vi "svl_Waterfall Display.vi"() -> ()   [LabVIEW 2017]
uses:
  <vilib>/addons/Sound and Vibration/compatibility/Waterfall/subVIs/svl_Waterfall Global.vi
panel:
  in  "palette":T1={"x axis width [%]"=80.0, "z axis height [%]"=40.0, "autoscale x"=FALSE, "autoscale y"=FALSE, "autoscale z max"=FALSE, "autoscale all"=FALSE, "transparency"=FALSE, "store view"=FALSE, "restore view"=FALSE} {"x axis width [%]" min=10.0 max=100.0 step=1.0 scale=10.0..100.0 scale format="%.1f"; "z axis height [%]" min=10.0 max=99.99 step=1.0 scale=10.0..100.0 scale format="%.1f"}
  in  "stop":bool
  in  "y axis":dbl(slide)=1234.0 scale=0.0..50.0 scale format="%.1f"
  in  "z axis":dbl(slide) scale format="%.1f"
  in  "x axis":dbl(slide) scale=0.0..30000.0 scale format="%.1f"
  out "Graph":cluster{dbl[], dbl[]}[](graph)
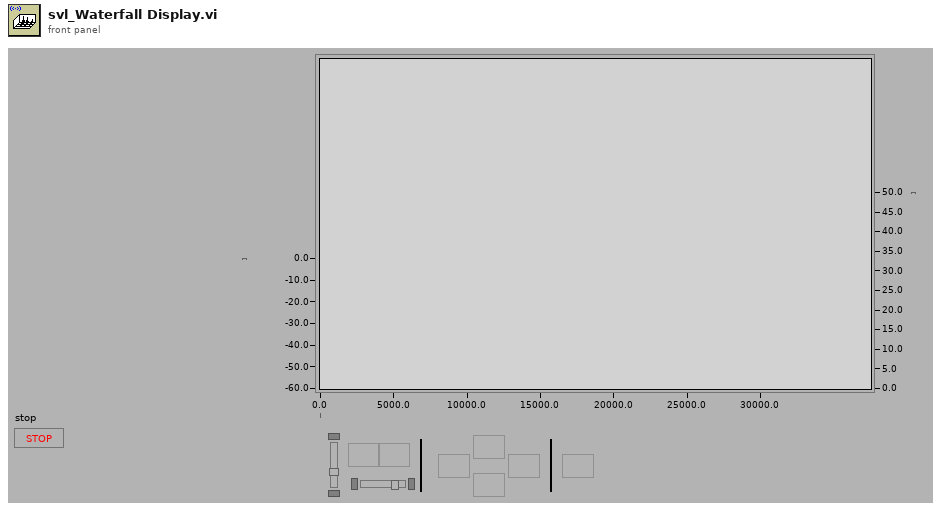
[diagram p1: front panel]
types:
  T1 = cluster{"x axis width [%]":dbl, "z axis height [%]":dbl, "autoscale x":bool, "autoscale y":bool, "autoscale z max":bool, "autoscale all":bool, "transparency":bool, "store view":bool, "restore view":bool}
  T2 = cluster{"autoscale x":bool, "autoscale y":bool, "autoscale z":bool, "autoscale all":bool, "transparency":bool, "store view":bool, "restore view":bool}
  T3 = cluster{"x axis width [%]":dbl, "z axis height [%]":dbl, "x axis minimum":dbl, "x axis maximum":dbl, "z axis minimum":dbl, "z axis maximum":dbl, "y axis minimum":dbl, "y axis maximum":dbl}
  T4 = typedef "LVPositionTypeDef.ctl" = cluster{"Left":i32, "Top":i32}
  T5 = cluster{"x axis width [%]":dbl, "z axis height [%]":dbl, "Scale.Minimum":dbl, "Scale.Maximum":dbl, "Scale.Minimum":dbl, "Scale.Maximum":dbl, "Scale.Minimum":dbl, "Scale.Maximum":dbl}
  T6 = cluster{"autoscale x":bool, "autoscale y":bool, "autoscale z max":bool, "autoscale all":bool, "transparency":bool, "store view":bool, "restore view":bool}
  T7 = cluster{"x axis width [%]":bool, "z axis height [%]":bool, bool, bool, bool, bool, bool, bool}
  T8 = cluster{"autoscale x":bool, "autoscale y":bool, bool, "autoscale all":bool, "transparency":bool, "store view":bool, "restore view":bool}
  T9 = cluster{"x axis width [%]":dbl, "z axis height [%]":dbl, "Scale.Minimum":dbl, "Scale.Maximum":dbl, "Scale.Minimum":dbl, "Scale.Maximum":dbl, "Scale.Minimum":dbl, "Scale.Maximum":dbl, "transparency":bool}
  T10 = cluster{"x axis":string, "y axis":string, "z axis":string}
  T11 = cluster{"Scale.Minimum":dbl, "Scale.Maximum":dbl}
  T12 = cluster{"y index":i32, "y length":i32, "x index":i32, "x length":i32}
  T13 = cluster{"frame":u32, "plot":u32, "background":u32}
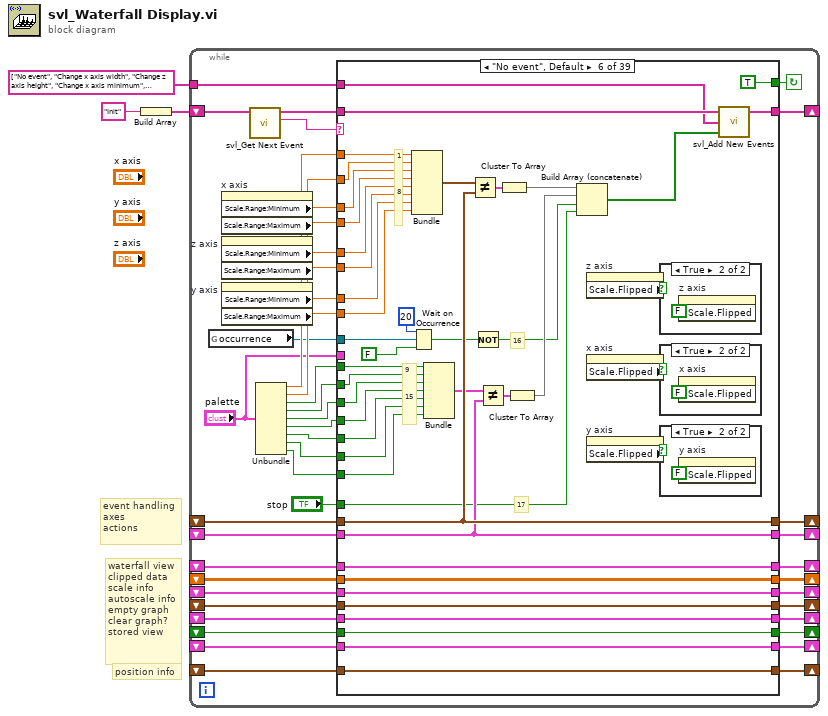
[diagram p0: block diagram]
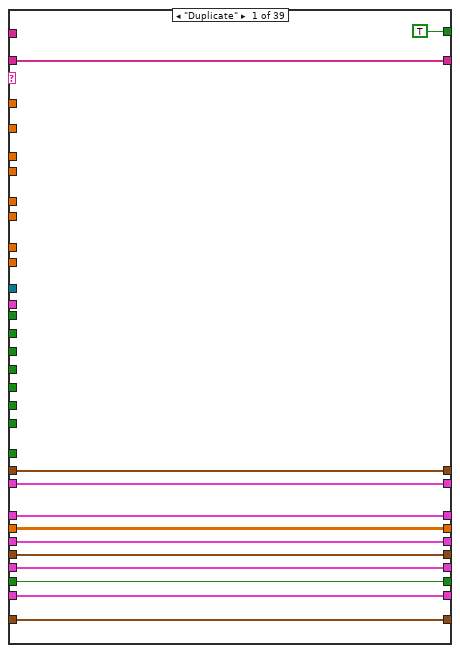
[diagram p2: hidden frame]
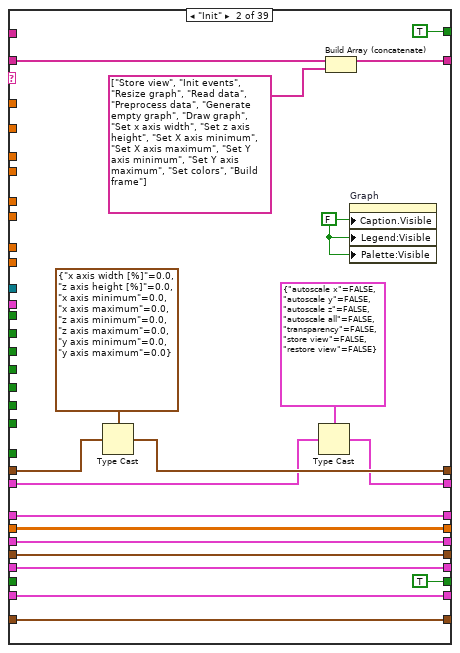
[diagram p3: hidden frame]
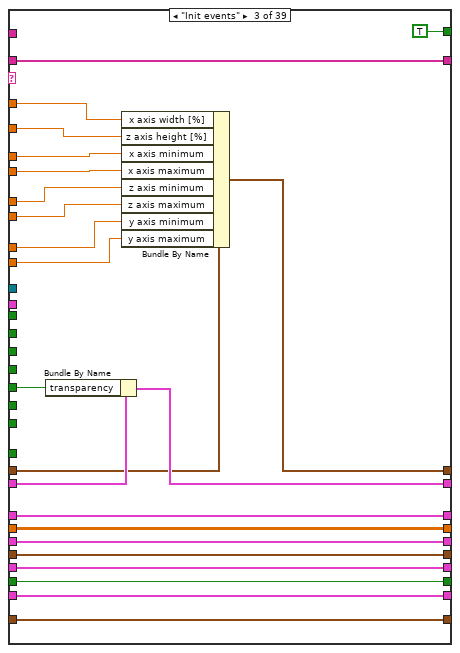
[diagram p4: hidden frame]
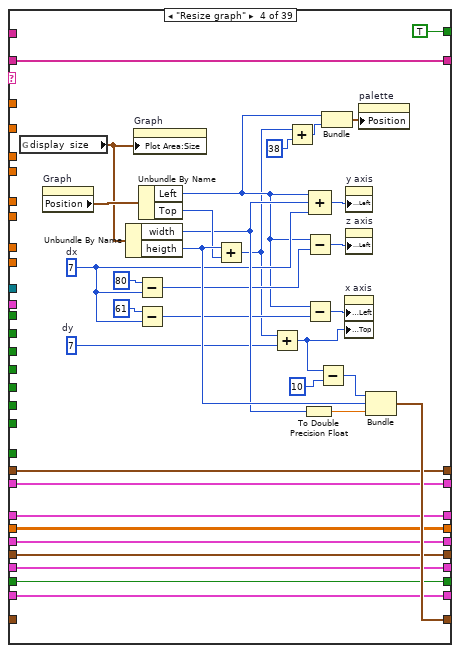
[diagram p5: hidden frame]
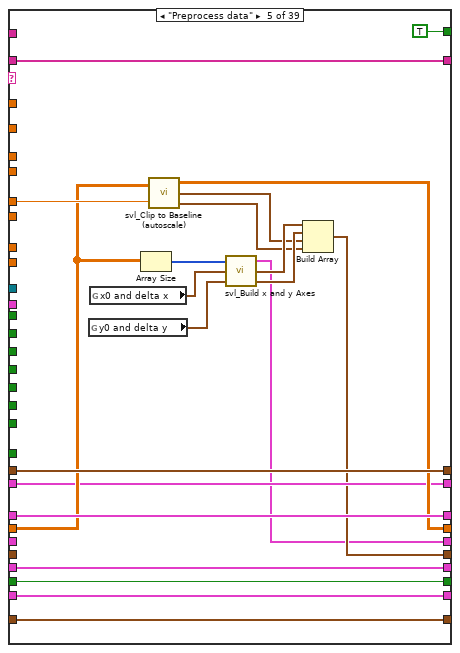
[diagram p6: hidden frame]
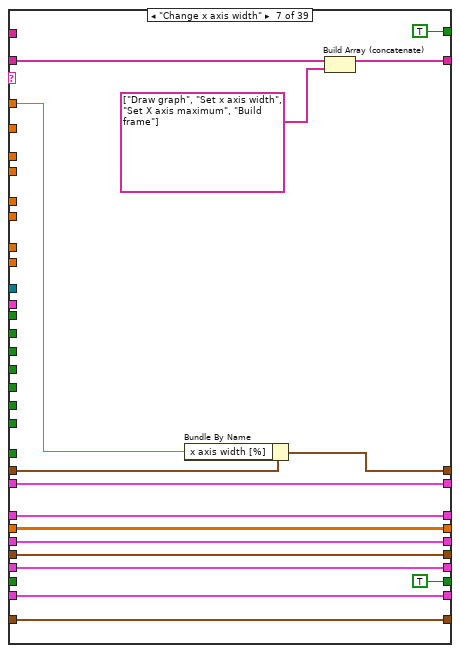
[diagram p10: hidden frame]
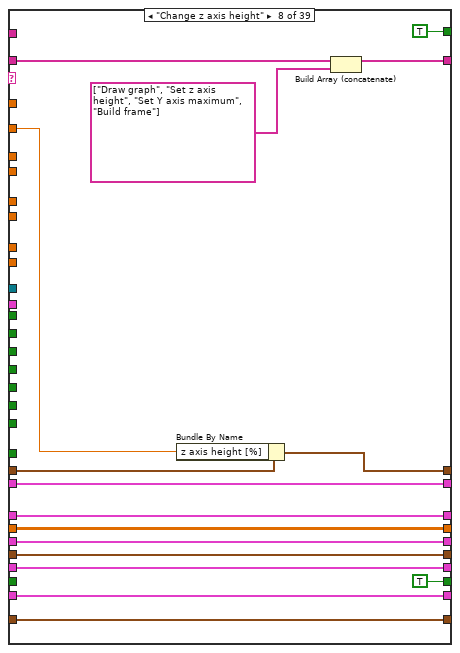
[diagram p11: hidden frame]
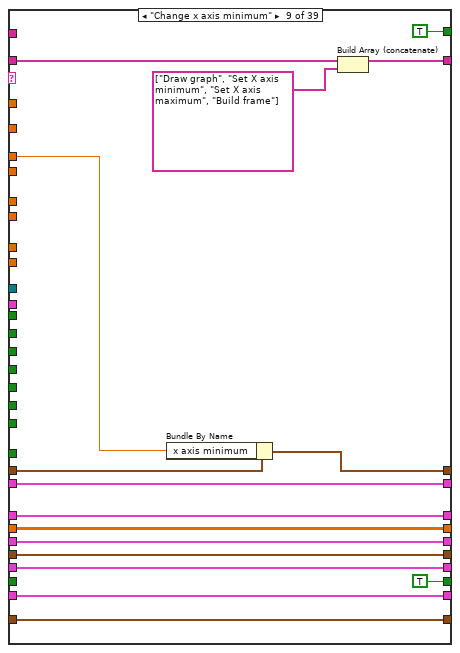
[diagram p12: hidden frame]
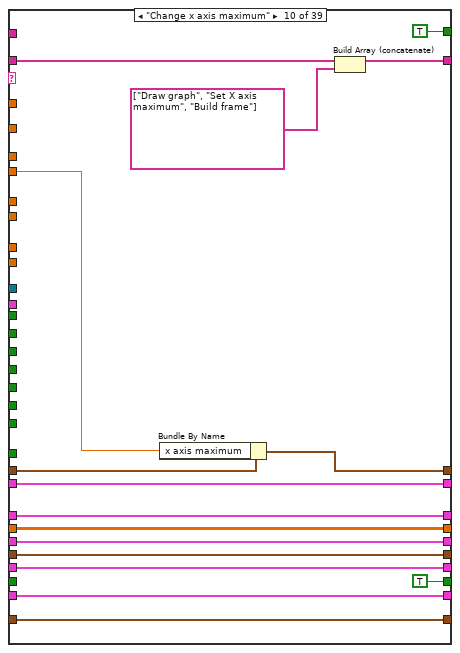
[diagram p13: hidden frame]
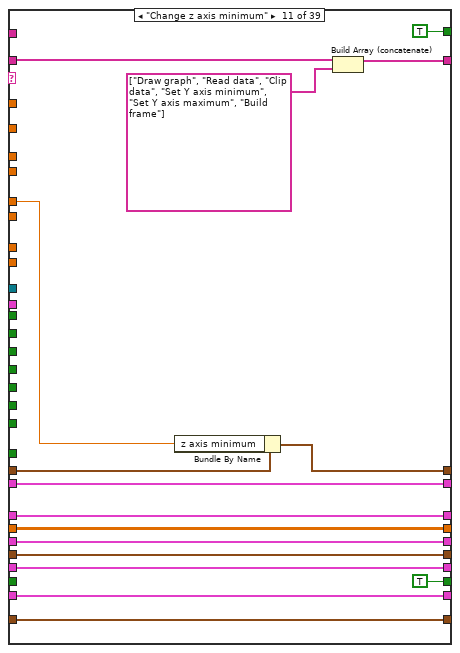
[diagram p14: hidden frame]
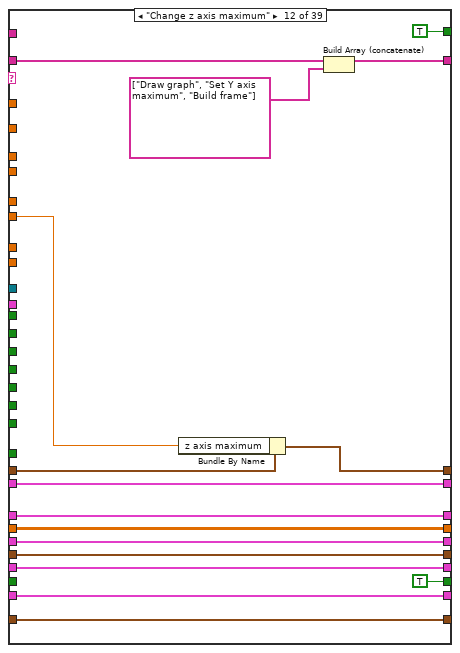
[diagram p15: hidden frame]
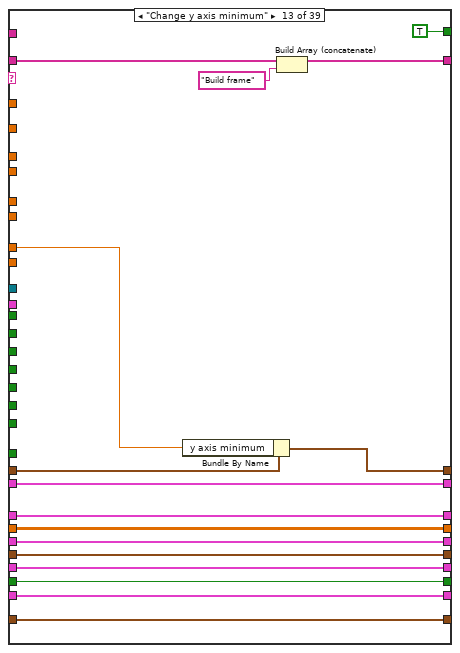
[diagram p16: hidden frame]
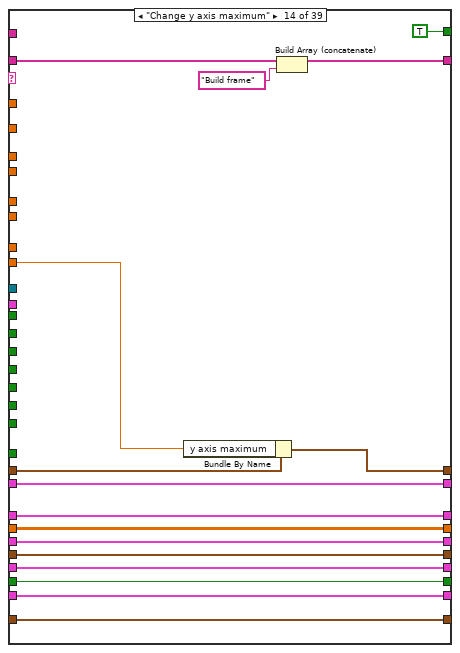
[diagram p17: hidden frame]
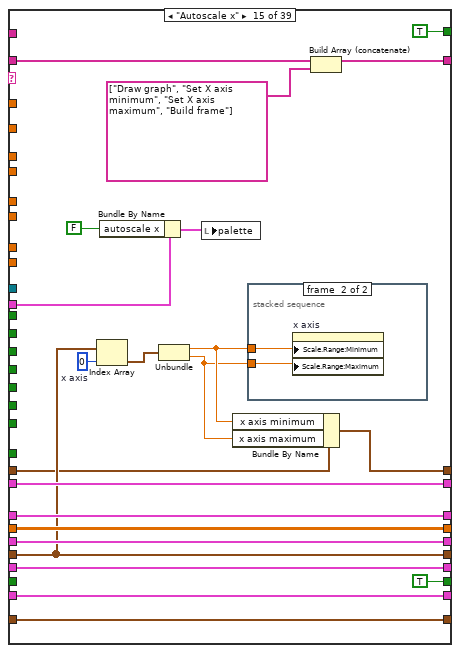
[diagram p18: hidden frame]
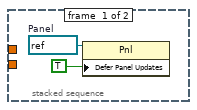
[diagram p19: hidden frame]
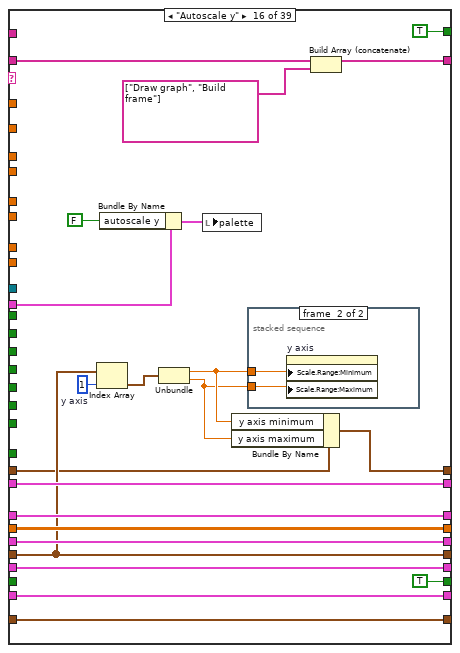
[diagram p20: hidden frame]
diagram:
  # "waterfall view\nclipped data\nscale info\nautoscale info\nempty graph\nclear graph?\nstored view"
  # "position info"
  # "event handling\naxes\nactions"
  n1 = Build Array("Init") -> (w2:string[])
  n2 = while {
    shift-left: _ -> [w16]
    shift-right: [w17] -> _
    shift-left: _ -> [w23]
    shift-right: [w22] -> _
    shift-left: _ -> [w25]
    shift-right: [w24] -> _
    shift-left: _ -> [w26]
    shift-right: [w27] -> _
    shift-left: _ -> [w29]
    shift-right: [w30] -> _
    shift-left: _ -> [w19]
    shift-right: [w32] -> _
    shift-left: _ -> [w31]
    shift-right: [w33] -> _
    shift-left: _ -> [w34]
    shift-right: [w35] -> _
    shift-left: _ -> [w38]
    shift-right: [w37] -> _
    shift-left: _ -> [w43]
    shift-right: [w44] -> _
    tunnel: string[] ["No event", "Change x axis width", "Change z axis height", "Change x axis minimum", "Change x axis maximum", "Change z axis minimum", "Change z axis maximum", "Change y axis minimum", "Change y axis maximum", "Autoscale x", "Autoscale y", "Autoscale z max", "Autoscale all", "Change transparency", "Store view", "Restore view", "Refresh", "Stop"] ("Event Names") -> [w46]
    shift-left: w2 -> [w21]
    shift-right: [w47] -> _
    stop <- w45 continue-if-true
    n3 = global read "svl_Waterfall Global.vi" "occurrence"() -> (w5:refnum<k4>)
    n4 = property on="x axis" class="Slide (strict)"() -> ("Scale.Range:Minimum"=w42:dbl, "Scale.Range:Maximum"=w41:dbl)  [unwired: 2 in, 2 out]
    n5 = property on="z axis" class="Slide (strict)"() -> ("Scale.Range:Minimum"=w40:dbl, "Scale.Range:Maximum"=w39:dbl)  [unwired: 2 in, 2 out]
    n6 = property on="y axis" class="Slide (strict)"() -> ("Scale.Range:Minimum"=w36:dbl, "Scale.Range:Maximum"=w28:dbl)  [unwired: 2 in, 2 out]
    n7 = call <vilib>:"svl_Get Next Event.vi"("Event Queue In"=w21) -> ("Next Event"=w4:string, "Event Queue Out"=w20:string[])  [unwired: 5 in]
    n8 = Unbundle("palette") -> ("x axis width [%]"=w15:dbl, "z axis height [%]"=w14:dbl, "autoscale x"=w7:bool, "autoscale y"=w8:bool, "autoscale z max"=w9:bool, "autoscale all"=w10:bool, "transparency"=w11:bool, "store view"=w12:bool, "restore view"=w13:bool)
    n9 = case shown="\"No event\", Default" w4 {
      tunnel: w20 -> [w58 w77 w93 w115 w156 w202 w220 w236 w251 w267 w283 w299 w306 w321 w343 w369 w393 w417 w433 w465 w474 w505 w526 w534 w570 w591 w631 w637 w654 w679 w696 w729 w751 w769 w800 w818 w823 w860 w887]
      tunnel: [w58 w76 w93 w115 w156 w201 w219 w222 w250 w254 w282 w298 w307 w322 w344 w360 w394 w418 w432 w465 w475 w504 w526 w534 w570 w591 w631 w637 w654 w679 w696 w729 w751 w769 w801 w818 w823 w860 w887] -> w47
      tunnel: w46 -> [_ _ _ _ _ w199 _ _ _ _ _ _ _ _ _ _ _ _ _ _ _ _ _ _ _ _ _ _ _ _ _ _ _ _ _ _ _ _ _]
      tunnel: [TRUE TRUE TRUE TRUE TRUE TRUE TRUE TRUE TRUE TRUE TRUE TRUE TRUE TRUE TRUE TRUE TRUE TRUE TRUE TRUE TRUE TRUE FALSE TRUE TRUE TRUE TRUE TRUE TRUE TRUE TRUE TRUE TRUE TRUE TRUE TRUE TRUE TRUE TRUE] -> w45
      tunnel: [w57 w72 w100 w125 w155 w197 w209 w225 w252 w268 w284 w300 w316 w332 w354 w380 w405 w425 w441 w464 w491 w513 w524 w556 w583 w602 w630 w648 w673 w690 w714 w728 w750 w768 w804 w817 w831 w871 w893] -> w44
      tunnel: w43 -> [w57 w72 w100 _ w155 w197 w209 w225 w252 w268 w284 w300 w316 w332 w354 w380 w405 w425 w441 w464 w491 w513 w524 w556 w583 w602 w630 w648 w673 w690 w714 w728 w750 w768 w804 w817 w831 w871 w893]
      tunnel: w15 -> [_ _ w84 _ _ w189 w210 _ _ _ _ _ _ _ _ _ _ _ _ w455 _ _ _ _ w578 _ _ _ w670 _ _ _ _ _ _ _ _ _ _]
      tunnel: w14 -> [_ _ w85 _ _ w196 _ w226 _ _ _ _ _ _ _ _ _ _ _ w454 _ _ _ _ _ w601 _ _ _ _ w707 _ _ _ w776 _ _ _ _]
      tunnel: w42 -> [_ _ w90 _ _ w195 _ _ w241 _ _ _ _ _ _ _ _ _ _ w453 _ _ _ _ _ _ _ w639 w672 _ _ _ _ _ w780 _ _ _ _]
      tunnel: w41 -> [_ _ w91 _ _ w190 _ _ _ w258 _ _ _ _ _ _ _ _ _ w452 _ _ _ _ _ _ _ _ w662 _ _ _ _ _ w774 _ _ _ _]
      tunnel: w40 -> [_ _ w89 _ w152 w194 _ _ _ _ w273 _ _ _ _ _ _ _ _ w451 _ _ _ _ _ _ _ _ _ w687 w706 _ w734 _ w778 _ _ _ _]
      tunnel: w39 -> [_ _ w88 _ _ w193 _ _ _ _ _ w291 _ _ _ _ _ _ _ w450 _ _ _ _ _ _ _ _ _ _ w705 _ _ _ w779 _ _ _ _]
      tunnel: [w56 w74 w80 w117 w154 w187 w218 w234 w242 w259 w276 w288 w308 w324 w342 w368 w396 w414 w440 w463 w490 w502 w523 w548 w579 w599 w621 w646 w664 w688 w697 w727 w743 w767 w802 w816 w830 w870 w892] -> w37
      tunnel: w38 -> [w56 w73 w81 w117 w154 w187 w217 w235 w243 w260 w275 w289 w309 w325 w341 w367 w395 w414 w440 w463 w490 w501 w523 w547 w577 w600 w621 w647 w663 w689 w697 w727 w742 w767 w802 w816 w830 w870 w892]
      tunnel: w36 -> [_ _ w87 _ _ w186 _ _ _ _ _ _ w303 _ _ _ _ _ _ w449 _ _ _ _ _ _ _ _ _ _ _ _ _ _ w788 _ _ _ _]
      tunnel: [w55 w71 w99 w116 w153 w184 w216 w233 w249 w266 w281 w297 w315 w331 w353 w379 w404 w424 w439 w462 w489 w512 w522 w555 w576 w598 w629 w645 w661 w686 w704 w726 w749 w766 w799 w811 w821 w857 w885] -> w35
      tunnel: w34 -> [w55 w71 w99 w116 w153 w184 w216 w233 w249 w266 w281 w297 w315 w331 w353 w379 w404 w424 w439 w462 w489 w512 w522 w555 w576 w598 w629 w645 w661 w686 w704 w726 w749 w766 _ w811 w821 w857 w885]
      tunnel: [w54 w70 w98 w114 w148 w183 w215 w232 w248 w265 w280 w296 w314 w330 w352 w378 w403 w423 w438 w461 w488 w511 w521 w554 w575 w597 w628 w644 w660 w685 w703 w719 w744 w756 w797 w815 w829 w869 w881] -> w33
      tunnel: [w53 w69 w97 w113 w143 w182 w214 w231 w247 w264 w272 w295 w313 w329 w348 w374 w399 w415 w437 w460 w487 w510 w520 w538 w574 w596 w627 w643 w659 w684 w702 w723 w732 w761 w798 w814 w828 w868 w891] -> w32
      tunnel: w31 -> [w54 w70 w98 w114 w145 w183 w215 w232 w248 w265 w280 w296 w314 w330 w352 w378 w403 w423 w438 w461 w488 w511 w521 w554 w575 w597 w628 w644 w660 w685 w703 _ w747 w756 w797 w815 w829 w869 w881]
      tunnel: w19 -> [w53 w69 w97 w113 _ w182 w214 w231 w247 w264 w272 w295 w313 w329 w348 w374 w399 w415 w437 w460 w487 w510 w520 w538 w574 w596 w627 w643 w659 w684 w702 w723 w733 w761 w798 w814 w828 w868 w891]
      tunnel: [w52 w68 w96 w112 w142 w181 w213 w230 w246 w263 w279 w294 w312 w328 w351 w377 w402 w422 w436 w459 w486 w509 w519 w553 w573 w595 w626 w642 w658 w683 w701 w722 w746 w762 w791 w813 w827 w867 w890] -> w30
      tunnel: w29 -> [w52 w68 w96 w112 _ w181 w213 w230 w246 w263 w279 w294 w312 w328 w351 w377 w402 w422 w436 w459 w486 w509 w519 w553 w573 w595 w626 w642 w658 w683 w701 w722 w746 w762 w791 w813 w827 w867 w890]
      tunnel: w28 -> [_ _ w86 _ _ w185 _ _ _ _ _ _ _ w323 _ _ _ _ _ w448 _ _ _ _ _ _ _ _ _ _ _ _ _ _ w789 _ _ _ _]
      tunnel: [w51 w67 w95 w111 w137 w180 w212 w229 w245 w262 w278 w293 w311 w327 w350 w376 w401 w421 w435 w458 w485 w508 w518 w552 w572 w594 w625 w641 w657 w682 w700 w724 w745 w765 w794 w812 w820 w856 w884] -> w27
      tunnel: w26 -> [w51 w67 w95 w111 w137 w180 w212 w229 w245 w262 w278 w293 w311 w327 w350 w376 w401 w421 w435 w458 w485 w508 w518 w552 w572 w594 w625 w641 w657 w682 w700 w724 w745 _ w794 w812 w820 w856 w884]
      tunnel: w25 -> [w50 _ w94 w110 w146 w179 _ _ _ _ _ _ w310 w326 _ _ _ _ _ w457 _ _ w517 w535 w569 w592 w624 w640 w656 w681 w699 w725 w748 w757 _ w808 w826 w866 w889]
      tunnel: [w50 TRUE w94 w110 w146 w179 TRUE TRUE TRUE TRUE TRUE TRUE w310 w326 TRUE TRUE TRUE TRUE TRUE w457 TRUE w503 w517 w535 w569 w592 w624 w640 w656 w681 w699 w725 w748 w757 FALSE FALSE w826 w866 w889] -> w24
      tunnel: w11 -> [_ _ w92 _ _ w174 _ _ _ _ _ _ _ _ _ _ _ _ w431 w447 _ _ _ _ _ _ _ _ _ _ _ _ _ _ _ _ w824 w861 _]
      tunnel: w23 -> [w49 w65 w83 w109 w144 w170 w211 w227 w240 w257 w274 w290 w305 w320 w349 w375 w400 w420 w430 w456 w484 w507 w516 w551 w571 w593 w623 w638 w655 w680 w698 w721 w741 w764 w785 w807 w825 w862 w888]
      tunnel: [w49 w66 w82 w109 w144 w170 w211 w227 w240 w257 w274 w290 w305 w320 w349 w375 w400 w420 w429 w456 w484 w507 w516 w551 w571 w593 w623 w638 w655 w680 w698 w721 w741 w764 w785 w807 w825 w862 w888] -> w22
      tunnel: w7 -> [_ _ _ _ _ w178 _ _ _ _ _ _ _ _ _ _ _ _ _ _ _ _ _ _ _ _ _ _ _ _ _ _ _ _ _ _ _ _ _]
      tunnel: w8 -> [_ _ _ _ _ w177 _ _ _ _ _ _ _ _ _ _ _ _ _ _ _ _ _ _ _ _ _ _ _ _ _ _ _ _ _ _ _ _ _]
      tunnel: w9 -> [_ _ _ _ _ w176 _ _ _ _ _ _ _ _ _ _ _ _ _ _ _ _ _ _ _ _ _ _ _ _ _ _ _ _ _ _ _ _ _]
      tunnel: w10 -> [_ _ _ _ _ w175 _ _ _ _ _ _ _ _ _ _ _ _ _ _ _ _ _ _ _ _ _ _ _ _ _ _ _ _ _ _ _ _ _]
      tunnel: "stop" -> [_ _ _ _ _ w163 _ _ _ _ _ _ _ _ _ _ _ _ _ _ _ _ _ _ _ _ _ _ _ _ _ _ _ _ _ _ _ _ _]
      tunnel: w12 -> [_ _ _ _ _ w169 _ _ _ _ _ _ _ _ _ _ _ _ _ _ _ _ _ _ _ _ _ _ _ _ _ _ _ _ _ _ _ _ _]
      tunnel: w13 -> [_ _ _ _ _ w168 _ _ _ _ _ _ _ _ _ _ _ _ _ _ _ _ _ _ _ _ _ _ _ _ _ _ _ _ _ _ _ _ _]
      tunnel: [w48 w62 w79 w108 w140 w167 w207 w224 w239 w256 w271 w287 w304 w319 w338 w364 w390 w416 w428 w446 w483 w506 w515 w536 w568 w590 w622 w636 w653 w678 w695 w720 w731 w763 w784 w806 w822 w859 w886] -> w17
      tunnel: w16 -> [w48 w62 w79 w108 w140 w167 w207 w224 w239 w256 w271 w287 w304 w319 w338 w364 w390 w416 w428 _ w483 w506 w515 w536 w568 w590 w622 w636 w653 w678 w695 w720 w731 w763 w784 w806 w822 w859 w886]
      tunnel: w5 -> [_ _ _ _ _ w160 _ _ _ _ _ _ _ _ _ _ _ _ _ _ _ _ _ _ _ _ _ _ _ _ _ _ _ _ _ _ _ _ _]
      tunnel: "palette" -> [_ _ _ _ _ _ _ _ _ _ _ _ _ _ w336 w361 w387 w411 _ w443 w473 _ _ _ _ _ _ _ _ _ _ _ _ _ _ _ _ _ _]
      frame "Duplicate" {
      }
      frame "Init" {
        w61 = FALSE ("Caption Visible")
        n10 = Type Cast(type=T3 {"x axis width [%]"=0.0, "z axis height [%]"=0.0, "x axis minimum"=0.0, "x axis maximum"=0.0, "z axis minimum"=0.0, "z axis maximum"=0.0, "y axis minimum"=0.0, "y axis maximum"=0.0}, x=w73) -> (*(type *) &x=w74:T3)
        n11 = Type Cast(type=T2 {"autoscale x"=FALSE, "autoscale y"=FALSE, "autoscale z"=FALSE, "autoscale all"=FALSE, "transparency"=FALSE, "store view"=FALSE, "restore view"=FALSE}, x=w65) -> (*(type *) &x=w66:T2)
        n12 = Build Array (concatenate)(w77, string[] ["Store view", "Init events", "Resize graph", "Read data", "Preprocess data", "Generate empty graph", "Draw graph", "Set x axis width", "Set z axis height", "Set X axis minimum", "Set X axis maximum", "Set Y axis minimum", "Set Y axis maximum", "Set colors", "Build frame"]) -> (w76:string[])
        n13 = property on="Graph" class="XYGraph (strict)"("Caption.Visible"=w61, "Legend:Visible"=w61, "Palette:Visible"=w61) -> ()  [unwired: 2 in, 2 out]
      }
      frame "Init events" {
        n14 = Bundle By Name(cluster=w83, "transparency"=w92) -> (w82:T2)
        n15 = Bundle By Name(cluster=w81, "x axis width [%]"=w84, "z axis height [%]"=w85, "x axis minimum"=w90, "x axis maximum"=w91, "z axis minimum"=w89, "z axis maximum"=w88, "y axis minimum"=w87, "y axis maximum"=w86) -> (w80:T3)
      }
      frame "Resize graph" {
        w119 = u32 7  # dx
        w118 = u32 7  # dy
        n16 = global read "svl_Waterfall Global.vi" "display  size"() -> (w102:cluster{"width":u32, "heigth":u32})
        n17 = property on="Graph" class="XYGraph (strict)"() -> ("Position"=w126:T4)  [unwired: 2 in, 2 out]
        n18 = Unbundle By Name(w102) -> ("width"=w130:u32, "heigth"=w135:u32)
        n19 = property on="Graph" class="XYGraph (strict)"("Plot Area:Size"=w102) -> ()  [unwired: 2 in, 2 out]
        n20 = Subtract(x=u32 80, y=w119) -> (x-y=w123:u32)
        n21 = Subtract(x=u32 61, y=w119) -> (x-y=w121:u32)
        n22 = Unbundle By Name(w126) -> ("Left"=w106:i32, "Top"=w132:i32)
        n23 = Add(x=w135, y=w132) -> (x+y=w105:u32)
        n24 = Add(x=w105, y=w118) -> (x+y=w120:u32)
        n25 = Add(x=w105, y=u32 38) -> (x+y=w103:u32)
        n26 = To Double Precision Float(number=w130) -> (double precision float=w134:dbl)
        n27 = Subtract(x=w106, y=w123) -> (x-y=w129:u32)
        n28 = Subtract(x=w106, y=w121) -> (x-y=w127:u32)
        n29 = Compound Arithmetic op=ADD(w106, w130, w119) -> (w128:u32)
        n30 = Subtract(x=w120, y=u32 10) -> (x-y=w133:u32)
        n31 = Bundle("Left"=w106, w103) -> (w107:cluster{"Left":i32, u32})  [unwired: 1 in]
        n32 = property on="x axis" class="Slide (strict)"("Position:Left"=w127, "Position:Top"=w120) -> ()  [unwired: 2 in, 2 out]
        n33 = property on="y axis" class="Slide (strict)"("Position:Left"=w128) -> ()  [unwired: 2 in, 2 out]
        n34 = property on="z axis" class="Slide (strict)"("Position:Left"=w129) -> ()  [unwired: 2 in, 2 out]
        n35 = property on="palette" class="Clust (strict)"("Position"=w107) -> ()  [unwired: 2 in, 2 out]
        n36 = Bundle(w133, "heigth"=w135, w134) -> (w125:cluster{u32, "heigth":u32, dbl})  [unwired: 1 in]
      }
      frame "Preprocess data" {
        n37 = global read "svl_Waterfall Global.vi" "y0 and delta y"() -> (w138:cluster{"y0":dbl, "delta y":dbl})
        n38 = global read "svl_Waterfall Global.vi" "x0 and delta x"() -> (w139:cluster{"x0":dbl, "delta x":dbl})
        n39 = Array Size(array=w145) -> (size(s)=w147:i32[])
        n40 = call <vilib>:"svl_Clip to Baseline (autoscale).vi"("waterfall data"=w145, "baseline"=w152) -> ("clipped data"=w148:dbl[][], "z autoscale"=w149:cluster{"z min":dbl, "z max":dbl}, "z scale"=w141:cluster{"z min":dbl, "z max":dbl})
        n41 = call <vilib>:"svl_Build x and y Axes.vi"("y0 and delta y"=w138, "x0 and delta x"=w139, "size(s)"=w147) -> ("y autoscale"=w150:cluster{"y min":dbl, "y max":dbl}, "x autoscale"=w151:cluster{"x min":dbl, "x max":dbl}, "scale info"=w142:cluster{"x scale":dbl[], "y scale":dbl[]})
        n42 = Build Array(w151, w150, w149, w141) -> (w143:cluster{"z min":dbl, "z max":dbl}[])
      }
      frame "No event", Default {
        # "16"
        # "17"
        # "9\n   \n\n15"
        # "1\n \n \n \n8"
        n43 = Wait on Occurrence(1:FALSE ("ignore previous (T)"), 2:w160, 3:20 ("ms timeout (-1)")) -> (0:w158:bool)
        n44 = Bundle("x axis width [%]"=w189, "z axis height [%]"=w196, "Scale.Minimum"=w195, "Scale.Maximum"=w190, "Scale.Minimum"=w194, "Scale.Maximum"=w193, "Scale.Minimum"=w186, "Scale.Maximum"=w185) -> (w192:T5)  [unwired: 1 in]
        n45 = Bundle("autoscale x"=w178, "autoscale y"=w177, "autoscale z max"=w176, "autoscale all"=w175, "transparency"=w174, "store view"=w169, "restore view"=w168) -> (w171:T6)  [unwired: 1 in]
        n46 = Not Equal?(x=w192, y=w187) -> (x != y?=w191:T7)
        n47 = Not(x=w158) -> (.not. x?=w162:bool)
        n48 = Not Equal?(x=w171, y=w170) -> (x != y?=w173:T8)
        n49 = Cluster To Array(cluster=w191) -> (array=w188:bool[])
        n50 = Cluster To Array(cluster=w173) -> (array=w172:bool[])
        n51 = Build Array (concatenate)(w188, w172, w162, w163) -> (w200:bool[])
        n52 = property on="z axis" class="Slide (strict)"() -> ("Scale.Flipped"=w166:bool)  [unwired: 2 in, 2 out]
        n53 = property on="x axis" class="Slide (strict)"() -> ("Scale.Flipped"=w165:bool)  [unwired: 2 in, 2 out]
        n54 = property on="y axis" class="Slide (strict)"() -> ("Scale.Flipped"=w164:bool)  [unwired: 2 in, 2 out]
        n55 = case shown="True" w166 {
          frame False {
          }
          frame True {
            n56 = property on="z axis" class="Slide (strict)"("Scale.Flipped"=FALSE ("Flipped")) -> ()  [unwired: 2 in, 2 out]
          }
        }
        n57 = case shown="True" w165 {
          frame False {
          }
          frame True {
            n58 = property on="x axis" class="Slide (strict)"("Scale.Flipped"=FALSE ("Flipped")) -> ()  [unwired: 2 in, 2 out]
          }
        }
        n59 = case shown="True" w164 {
          frame False {
          }
          frame True {
            n60 = property on="y axis" class="Slide (strict)"("Scale.Flipped"=FALSE ("Flipped")) -> ()  [unwired: 2 in, 2 out]
          }
        }
        n61 = call <vilib>:"svl_Add New Events.vi"("New Events"=w200, "Event Names"=w199, "Event Queue In"=w202) -> ("Event Queue Out"=w201:string[])  [unwired: 2 in]
      }
      frame "Change x axis width" {
        n62 = Bundle By Name(cluster=w217, "x axis width [%]"=w210) -> (w218:T3)
        n63 = Build Array (concatenate)(w220, string[] ["Draw graph", "Set x axis width", "Set X axis maximum", "Build frame"]) -> (w219:string[])
      }
      frame "Change z axis height" {
        n64 = Bundle By Name(cluster=w235, "z axis height [%]"=w226) -> (w234:T3)
        n65 = Build Array (concatenate)(w236, string[] ["Draw graph", "Set z axis height", "Set Y axis maximum", "Build frame"]) -> (w222:string[])
      }
      frame "Change x axis minimum" {
        n66 = Bundle By Name(cluster=w243, "x axis minimum"=w241) -> (w242:T3)
        n67 = Build Array (concatenate)(w251, string[] ["Draw graph", "Set X axis minimum", "Set X axis maximum", "Build frame"]) -> (w250:string[])
      }
      frame "Change x axis maximum" {
        n68 = Bundle By Name(cluster=w260, "x axis maximum"=w258) -> (w259:T3)
        n69 = Build Array (concatenate)(w267, string[] ["Draw graph", "Set X axis maximum", "Build frame"]) -> (w254:string[])
      }
      frame "Change z axis minimum" {
        n70 = Bundle By Name(cluster=w275, "z axis minimum"=w273) -> (w276:T3)
        n71 = Build Array (concatenate)(w283, string[] ["Draw graph", "Read data", "Clip data", "Set Y axis minimum", "Set Y axis maximum", "Build frame"]) -> (w282:string[])
      }
      frame "Change z axis maximum" {
        n72 = Bundle By Name(cluster=w289, "z axis maximum"=w291) -> (w288:T3)
        n73 = Build Array (concatenate)(w299, string[] ["Draw graph", "Set Y axis maximum", "Build frame"]) -> (w298:string[])
      }
      frame "Change y axis minimum" {
        n74 = Bundle By Name(cluster=w309, "y axis minimum"=w303) -> (w308:T3)
        n75 = Build Array (concatenate)(w306, "Build frame") -> (w307:string[])
      }
      frame "Change y axis maximum" {
        n76 = Bundle By Name(cluster=w325, "y axis maximum"=w323) -> (w324:T3)
        n77 = Build Array (concatenate)(w321, "Build frame") -> (w322:string[])
      }
      frame "Autoscale x" {
        w347 = 0  # x axis
        n78 = Index Array(array=w348, index=w347) -> (element=w346:cluster{"z min":dbl, "z max":dbl})
        n79 = Bundle By Name(cluster=w336, "autoscale x"=FALSE) -> (w337:T1)
        n80 = Unbundle(w346) -> ("z min"=w340:dbl, "z max"=w339:dbl)
        n81 = local write "palette"(w337) -> ()
        n82 = Bundle By Name(cluster=w341, "x axis minimum"=w340, "x axis maximum"=w339) -> (w342:T3)
        n83 = stacked-sequence {
          tunnel: w340 -> [_ w359]
          tunnel: w339 -> [_ w358]
          frame #0 {
            w356 = refnum<vi> refnum  # Panel
            n84 = property class="Pnl"(reference=w356, "Defer Panel Updates"=TRUE) -> ()  [unwired: 1 in, 2 out]
          }
          frame #1 {
            n85 = property on="x axis" class="Slide (strict)"("Scale.Range:Minimum"=w359, "Scale.Range:Maximum"=w358) -> ()  [unwired: 2 in, 2 out]
          }
        }
        n86 = Build Array (concatenate)(w343, string[] ["Draw graph", "Set X axis minimum", "Set X axis maximum", "Build frame"]) -> (w344:string[])
      }
      frame "Autoscale y" {
        w373 = 1  # y axis
        n87 = Index Array(array=w374, index=w373) -> (element=w372:cluster{"z min":dbl, "z max":dbl})
        n88 = Bundle By Name(cluster=w361, "autoscale y"=FALSE ("autoscale x")) -> (w363:T1)
        n89 = Unbundle(w372) -> ("z min"=w366:dbl, "z max"=w365:dbl)
        n90 = local write "palette"(w363) -> ()
        n91 = Bundle By Name(cluster=w367, "y axis minimum"=w366, "y axis maximum"=w365) -> (w368:T3)
        n92 = stacked-sequence {
          tunnel: w366 -> [_ w385]
          tunnel: w365 -> [_ w384]
          frame #0 {
            w382 = refnum<vi> refnum  # Panel
            n93 = property class="Pnl"(reference=w382, "Defer Panel Updates"=TRUE) -> ()  [unwired: 1 in, 2 out]
          }
          frame #1 {
            n94 = property on="y axis" class="Slide (strict)"("Scale.Range:Minimum"=w385, "Scale.Range:Maximum"=w384) -> ()  [unwired: 2 in, 2 out]
          }
        }
        n95 = Build Array (concatenate)(w369, string[] ["Draw graph", "Build frame"]) -> (w360:string[])
      }
      frame "Autoscale z max" {
        w398 = 2  # z axis
        n96 = Bundle By Name(cluster=w387, "autoscale z max"=FALSE ("autoscale x")) -> (w389:T1)
        n97 = Index Array(array=w399, index=w398) -> (element=w392:cluster{"z min":dbl, "z max":dbl})
        n98 = Unbundle(w392) -> ("z max"=w391:dbl)  [unwired: 1 out]
        n99 = local write "palette"(w389) -> ()
        n100 = stacked-sequence {
          tunnel: w391 -> [_ w409]
          frame #0 {
            w407 = refnum<vi> refnum  # Panel
            n101 = property class="Pnl"(reference=w407, "Defer Panel Updates"=TRUE) -> ()  [unwired: 1 in, 2 out]
          }
          frame #1 {
            n102 = property on="z axis" class="Slide (strict)"("Scale.Range:Maximum"=w409) -> ()  [unwired: 2 in, 2 out]
          }
        }
        n103 = Bundle By Name(cluster=w395, "z axis maximum"=w391) -> (w396:T3)
        n104 = Build Array (concatenate)(w393, string[] ["Draw graph", "Set Y axis maximum", "Build frame"]) -> (w394:string[])
      }
      frame "Autoscale all" {
        n105 = Bundle By Name(cluster=w411, "autoscale all"=FALSE ("autoscale x")) -> (w413:T1)
        n106 = local write "palette"(w413) -> ()
        n107 = Build Array (concatenate)(w417, string[] ["Draw graph", "Set all scales", "Set X axis minimum", "Set X axis maximum", "Set Y axis maximum", "Build frame"]) -> (w418:string[])
      }
      frame "Change transparency" {
        n108 = Bundle By Name(cluster=w430, "transparency"=w431) -> (w429:T2)
        n109 = Build Array (concatenate)(w433, string[] ["Draw graph", "Set transparency", "Draw graph"]) -> (w432:string[])
      }
      frame "Store view" {
        n110 = Bundle By Name(cluster=w443, "store view"=FALSE ("autoscale x")) -> (w445:T1)
        n111 = Bundle("x axis width [%]"=w455, "z axis height [%]"=w454, "Scale.Minimum"=w453, "Scale.Maximum"=w452, "Scale.Minimum"=w451, "Scale.Maximum"=w450, "Scale.Minimum"=w449, "Scale.Maximum"=w448, "transparency"=w447) -> (w446:T9)  [unwired: 1 in]
        n112 = local write "palette"(w445) -> ()
      }
      frame "Restore view" {
        n113 = Unbundle(w483) -> ("x axis width [%]"=w471:dbl, "z axis height [%]"=w470:dbl, "Scale.Minimum"=w482:dbl, "Scale.Maximum"=w481:dbl, "Scale.Minimum"=w480:dbl, "Scale.Maximum"=w479:dbl, "Scale.Minimum"=w478:dbl, "Scale.Maximum"=w477:dbl, "transparency"=w469:bool)
        n114 = Bundle By Name(cluster=w473, "x axis width [%]"=w471, "z axis height [%]"=w470, "transparency"=w469, "restore view"=FALSE) -> (w472:T1)
        n115 = stacked-sequence {
          tunnel: w482 -> [_ w500]
          tunnel: w481 -> [_ w499]
          tunnel: w480 -> [_ w498]
          tunnel: w479 -> [_ w497]
          tunnel: w478 -> [_ w496]
          tunnel: w477 -> [_ w495]
          frame #0 {
            w493 = refnum<vi> refnum  # Panel
            n116 = property class="Pnl"(reference=w493, "Defer Panel Updates"=FALSE) -> ()  [unwired: 1 in, 2 out]
          }
          frame #1 {
            n117 = property on="x axis" class="Slide (strict)"("Scale.Range:Minimum"=w500, "Scale.Range:Maximum"=w499) -> ()  [unwired: 2 in, 2 out]
            n118 = property on="z axis" class="Slide (strict)"("Scale.Range:Minimum"=w498, "Scale.Range:Maximum"=w497) -> ()  [unwired: 2 in, 2 out]
            n119 = property on="y axis" class="Slide (strict)"("Scale.Range:Minimum"=w496, "Scale.Range:Maximum"=w495) -> ()  [unwired: 2 in, 2 out]
          }
        }
        n120 = local write "palette"(w472) -> ()
        n121 = Build Array (concatenate)(w474, string[] ["Draw graph", "Init events", "Read data", "Clip data", "Set x axis width", "Set z axis height", "Set X axis minimum", "Set X axis maximum", "Set Y axis minimum", "Set Y axis maximum", "Set transparency", "Build frame"]) -> (w475:string[])
      }
      frame "Refresh" {
        n122 = call <vilib>:"svl_Refresh.vi"("axes IN"=w501, "event queue IN"=w505) -> ("clear graph?"=w503:bool, "axes OUT"=w502:T3, "event queue OUT"=w504:string[])  [unwired: 1 in]
      }
      frame "Stop" {
      }
      frame "Set all scales" {
        w529 = " "  # non-breaking space (Alt 0160)
        w540 = 2  # z axis
        w544 = 1  # y axis
        w550 = 0  # x axis
        n123 = global read "svl_Waterfall Global.vi" "axis labels"() -> (w533:T10)
        n124 = Index Array(array=w538, index=w550) -> (element=w549:cluster{"z min":dbl, "z max":dbl})
        n125 = Index Array(array=w538, index=w540) -> (element=w539:cluster{"z min":dbl, "z max":dbl})
        n126 = Index Array(array=w538, index=w544) -> (element=w543:cluster{"z min":dbl, "z max":dbl})
        n127 = Unbundle(w533) -> ("x axis"=w532:string, "y axis"=w531:string, "z axis"=w530:string)
        n128 = Unbundle(w549) -> ("z min"=w546:dbl, "z max"=w545:dbl)
        n129 = Unbundle(w543) -> ("z min"=w542:dbl, "z max"=w541:dbl)
        n130 = Unbundle(w539) -> ("z max"=w537:dbl)  [unwired: 1 out]
        n131 = Concatenate Strings(w531, w529) -> (w528:string)
        n132 = Concatenate Strings(w530, w529) -> (w527:string)
        n133 = stacked-sequence {
          tunnel: w546 -> [_ w567]
          tunnel: w545 -> [_ w566]
          tunnel: w542 -> [_ w565]
          tunnel: w541 -> [_ w564]
          tunnel: w537 -> [_ w563]
          tunnel: w532 -> [_ w562]
          tunnel: w528 -> [_ w561]
          tunnel: w527 -> [_ w560]
          frame #0 {
            w558 = refnum<vi> refnum  # Panel
            n134 = property class="Pnl"(reference=w558, "Defer Panel Updates"=TRUE) -> ()  [unwired: 1 in, 2 out]
          }
          frame #1 {
            n135 = property on="x axis" class="Slide (strict)"("Scale.Range:Minimum"=w567, "Scale.Range:Maximum"=w566, "Caption.Text"=w562) -> ()  [unwired: 2 in, 2 out]
            n136 = property on="y axis" class="Slide (strict)"("Scale.Range:Minimum"=w565, "Scale.Range:Maximum"=w564, "Caption.Text"=w561) -> ()  [unwired: 2 in, 2 out]
            n137 = property on="z axis" class="Slide (strict)"("Scale.Range:Maximum"=w563, "Caption.Text"=w560) -> ()  [unwired: 2 in, 2 out]
          }
        }
        n138 = Bundle By Name(cluster=w547, "z axis maximum"=w537, "y axis minimum"=w542, "y axis maximum"=w541, "x axis minimum"=w546, "x axis maximum"=w545) -> (w548:T3)
      }
      frame "Set x axis width" {
        n139 = Unbundle(w583) -> (w582:dbl)  [unwired: 2 out]
        n140 = Compound Arithmetic op=MULTIPLY(w578, w582, 0.01) -> (w584:dbl)
        n141 = Bundle By Name(cluster=w577, "x axis width [%]"=w578) -> (w579:T3)
        n142 = Round Toward +Infinity(x=w584) -> (ceil(x): smallest int >= x=w580:dbl)
        n143 = To Unsigned Long Integer(number=w580) -> (unsigned 32bit integer=w585:u32)
        n144 = stacked-sequence {
          tunnel: w585 -> [_ w589]
          frame #0 {
            w587 = refnum<vi> refnum  # Panel
            n145 = property class="Pnl"(reference=w587, "Defer Panel Updates"=TRUE) -> ()  [unwired: 1 in, 2 out]
          }
          frame #1 {
            n146 = property on="x axis" class="Slide (strict)"("Housing Size:Width"=w589) -> ()  [unwired: 2 in, 2 out]
          }
        }
      }
      frame "Set z axis height" {
        n147 = stacked-sequence {
          tunnel: w602 -> [_ _ w610 _]
          tunnel: w601 -> [_ _ w608 _]
          frame #0 {
            w605 = refnum<vi> refnum  # Panel
            n148 = property class="Pnl"(reference=w605, "Defer Panel Updates"=TRUE) -> ()  [unwired: 1 in, 2 out]
          }
          frame #1 {
            w606 = FALSE ("Caption.Visible")
            n149 = property on="y axis" class="Slide (strict)"("Caption.Visible"=w606) -> ()  [unwired: 2 in, 2 out]
            n150 = property on="z axis" class="Slide (strict)"("Caption.Visible"=w606) -> ()  [unwired: 2 in, 2 out]
          }
          frame #2 {
            n151 = Unbundle(w610) -> (w617:u32, "heigth"=w618:u32)  [unwired: 1 out]
            n152 = To Double Precision Float(number=w618) -> (double precision float=w616:dbl)
            n153 = Compound Arithmetic op=MULTIPLY(w608, w616, 0.01) -> (w611:dbl)
            n154 = Round Toward +Infinity(x=w611) -> (ceil(x): smallest int >= x=w609:dbl)
            n155 = To Unsigned Long Integer(number=w609) -> (unsigned 32bit integer=w613:u32)
            n156 = Subtract(x=w618, y=w613) -> (x-y=w614:u32)
            n157 = Subtract(x=w617, y=w614) -> (x-y=w615:u32)
            n158 = Subtract(x=w617, y=w613) -> (x-y=w612:u32)
            n159 = property on="z axis" class="Slide (strict)"("Position:Top"=w612, "Housing Size:Height"=w613) -> ()  [unwired: 2 in, 2 out]
            n160 = property on="y axis" class="Slide (strict)"("Position:Top"=w615, "Housing Size:Height"=w614) -> ()  [unwired: 2 in, 2 out]
          }
          frame #3 {
            w619 = TRUE ("Caption.Visible")
            n161 = property on="y axis" class="Slide (strict)"("Caption.Visible"=w619) -> ()  [unwired: 2 in, 2 out]
            n162 = property on="z axis" class="Slide (strict)"("Caption.Visible"=w619) -> ()  [unwired: 2 in, 2 out]
          }
        }
        n163 = Bundle By Name(cluster=w600, "z axis height [%]"=w601) -> (w599:T3)
      }
      frame "Set z axis minimum" {
        n164 = Unbundle By Name(w621) -> ("z axis minimum"=w620:dbl)
        n165 = stacked-sequence {
          tunnel: w620 -> [_ w635]
          frame #0 {
            w633 = refnum<vi> refnum  # Panel
            n166 = property class="Pnl"(reference=w633, "Defer Panel Updates"=TRUE) -> ()  [unwired: 1 in, 2 out]
          }
          frame #1 {
            n167 = property on="z axis" class="Slide (strict)"("Scale.Range:Minimum"=w635) -> ()  [unwired: 2 in, 2 out]
          }
        }
      }
      frame "Set X axis minimum" {
        n168 = stacked-sequence {
          tunnel: w639 -> [_ w652]
          frame #0 {
            w650 = refnum<vi> refnum  # Panel
            n169 = property class="Pnl"(reference=w650, "Defer Panel Updates"=TRUE) -> ()  [unwired: 1 in, 2 out]
          }
          frame #1 {
            n170 = property on="Graph" class="XYGraph (strict)"("X Scale.Range:Minimum"=w652) -> ()  [unwired: 2 in, 2 out]
          }
        }
        n171 = Bundle By Name(cluster=w647, "x axis minimum"=w639) -> (w646:T3)
      }
      frame "Set X axis maximum" {
        n172 = Multiply(x=0.01, y=w670) -> (x*y=w668:dbl)
        n173 = Subtract(x=w662, y=w672) -> (x-y=w667:dbl)
        n174 = Reciprocal(x=w668) -> (1/x=w666:dbl)
        n175 = Multiply(x=w666, y=w667) -> (x*y=w665:dbl)
        n176 = Bundle By Name(cluster=w663, "x axis maximum"=w662) -> (w664:T3)
        n177 = Add(x=w665, y=w672) -> (x+y=w671:dbl)
        n178 = stacked-sequence {
          tunnel: w671 -> [_ w677]
          frame #0 {
            w676 = refnum<vi> refnum  # Panel
            n179 = property class="Pnl"(reference=w676, "Defer Panel Updates"=TRUE) -> ()  [unwired: 1 in, 2 out]
          }
          frame #1 {
            n180 = property on="Graph" class="XYGraph (strict)"("X Scale.Range:Maximum"=w677) -> ()  [unwired: 2 in, 2 out]
          }
        }
      }
      frame "Set Y axis minimum" {
        n181 = stacked-sequence {
          tunnel: w687 -> [_ w694]
          frame #0 {
            w692 = refnum<vi> refnum  # Panel
            n182 = property class="Pnl"(reference=w692, "Defer Panel Updates"=TRUE) -> ()  [unwired: 1 in, 2 out]
          }
          frame #1 {
            n183 = property on="Graph" class="XYGraph (strict)"("Y Scale.Range:Minimum"=w694) -> ()  [unwired: 2 in, 2 out]
          }
        }
        n184 = Bundle By Name(cluster=w689, "z axis minimum"=w687) -> (w688:T3)
      }
      frame "Set Y axis maximum" {
        n185 = Multiply(x=0.01, y=w707) -> (x*y=w711:dbl)
        n186 = Subtract(x=w705, y=w706) -> (x-y=w710:dbl)
        n187 = Reciprocal(x=w711) -> (1/x=w709:dbl)
        n188 = Multiply(x=w709, y=w710) -> (x*y=w708:dbl)
        n189 = Add(x=w708, y=w706) -> (x+y=w713:dbl)
        n190 = stacked-sequence {
          tunnel: w713 -> [_ w718]
          frame #0 {
            w716 = refnum<vi> refnum  # Panel
            n191 = property class="Pnl"(reference=w716, "Defer Panel Updates"=TRUE) -> ()  [unwired: 1 in, 2 out]
          }
          frame #1 {
            n192 = property on="Graph" class="XYGraph (strict)"("Y Scale.Range:Maximum"=w718) -> ()  [unwired: 2 in, 2 out]
          }
        }
      }
      frame "Read data" {
        n193 = global read "svl_Waterfall Global.vi" "waterfall data"() -> (w719:dbl[][])
      }
      frame "Clip data" {
        w740 = 3  # absolute z max
        w738 = 2  # z axis
        n194 = call <vilib>:"svl_Clip to Baseline.vi"("baseline"=w734, "waterfall data"=w747) -> ("clipped data"=w744:dbl[][])
        n195 = Index Array(array=w733, index=w740) -> (element=w739:cluster{"z min":dbl, "z max":dbl})
        n196 = Unbundle(w739) -> ("z max"=w737:dbl)  [unwired: 1 out]
        n197 = Bundle By Name(cluster=w742, "z axis minimum"=w734) -> (w743:T3)
        n198 = Bundle("Scale.Minimum"=w734, "z max"=w737) -> (w736:cluster{"Scale.Minimum":dbl, "z max":dbl})  [unwired: 1 in]
        n199 = call <vilib>:"svl_Autoscale.vi"("scale"=w736) -> ("autoscale"=w735:cluster{"min":dbl, "max":dbl})
        n200 = Replace Array Subset(array=w733, new element=w735, index=w738) -> (w732:cluster{"z min":dbl, "z max":dbl}[])
      }
      frame "Generate empty graph" {
        n201 = Array Size(array=w756) -> (size(s)=w755:i32[])
        n202 = Index Array(array=w755, index=0) -> (element=w754:i32)
        n203 = Add(x=w754, y=2) -> (x+y=w759:i32)
        n204 = Initialize Array(cluster{dbl[], dbl[]} {[nan], [nan]} ("frame"), w759) -> (w765:cluster{dbl[], dbl[]}[])
      }
      frame "Build frame" {
        w771 = refnum<vi> refnum  # Panel
        n205 = Bundle("Scale.Minimum"=w780, "Scale.Maximum"=w774) -> (w773:T11)  [unwired: 1 in]
        n206 = Bundle("Scale.Minimum"=w778, "Scale.Maximum"=w779) -> (w775:T11)  [unwired: 1 in]
        n207 = Bundle("Scale.Minimum"=w788, "Scale.Maximum"=w789) -> (w787:T11)  [unwired: 1 in]
        n208 = property on="Graph" class="XYGraph (strict)"() -> ("X Scale.Range:Maximum"=w777:dbl, "Y Scale.Range:Maximum"=w803:dbl)  [unwired: 2 in, 2 out]
        n209 = call <vilib>:"svl_Limit x and y Axes.vi"("y scale"=w787, "x scale"=w773, "scale info"=w791) -> ("subset info"=w786:T12, "scale subset"=w790:cluster{"x scale":dbl[], "y scale":dbl[]})
        n210 = call <vilib>:"svl_Compute Frame and Perspective.vi"("x scale"=w773, "z scale"=w775, "z axis height [%]"=w776, "X maximum"=w777, "Y maximum"=w803) -> ("front frame"=w781:cluster{dbl[], dbl[]}, "back frame"=w782:cluster{dbl[], dbl[]}, "dY"=w796:dbl, "dX/dY"=w795:dbl)  [unwired: 2 in]
        n211 = call <vilib>:"svl_Generate Waterfall View.vi"("scale info"=w790, "clipped data"=w797, "dX/dY"=w795, "dY"=w796, "y scale"=w787, "subset info"=w786) -> ("waterfall view"=w783:cluster{dbl[], dbl[]}[])
        n212 = property class="Pnl"(reference=w771, "Defer Panel Updates"=FALSE) -> ()  [unwired: 1 in, 2 out]
        n213 = Build Array (concatenate)(w800, "Draw graph") -> (w801:string[])
        n214 = Build Array (concatenate)(w781, w783, w782) -> (w799:cluster{dbl[], dbl[]}[])
      }
      frame "Draw graph" {
        n215 = Select(t=w812, s=w808, f=w811) -> (s? t:f=→"Graph":cluster{dbl[], dbl[]}[])
      }
      frame "Set transparency" {
        n216 = stacked-sequence {
          tunnel: w824 -> [_ w839 _]
          tunnel: w820 -> [_ w837 _]
          frame #0 {
            w834 = refnum<vi> refnum  # Panel
            n217 = property class="Pnl"(reference=w834, "Defer Panel Updates"=TRUE) -> ()  [unwired: 1 in, 2 out]
          }
          frame #1 {
            n218 = Array Size(array=w837) -> (size(s)=w838:i32)
            n219 = Decrement(x=w838) -> (x-1=w835:i32)
            n220 = Decrement(x=w835) -> (x-1=w836:i32)
            n221 = Select(t=i16 -1, s=w839, f=i16 -3 ("t")) -> (s? t:f=w840:i16)
            n222 = for {
              N: w836 -> [_]
              tunnel: w840 -> [w843]
              i -> [w845]
              n223 = Increment(x=w845) -> (x+1=w844:i32)
              n224 = property on="Graph" class="XYGraph (strict)"("Active Plot"=w844, "Plot.Fill To"=w843) -> ()  [unwired: 2 in, 2 out]
            }
          }
          frame #2 {
            w847 = refnum<vi> refnum  # Panel
            n225 = property class="Pnl"(reference=w847, "Defer Panel Updates"=FALSE) -> ()  [unwired: 1 in, 2 out]
          }
        }
      }
      frame "Set colors" {
        w855 = i16 -1 ("Fill To")
        n226 = global read "svl_Waterfall Global.vi" "colors"() -> (w849:T13)
        n227 = Array Size(array=w856) -> (size(s)=w858:i32)
        n228 = Unbundle By Name(w849) -> ("frame"=w851:u32)
        n229 = Unbundle By Name(w849) -> ("background"=w848:u32)
        n230 = Unbundle By Name(w849) -> ("plot"=w850:u32)
        n231 = Decrement(x=w858) -> (x-1=w854:i32)
        n232 = Select(t=i16 -1, s=w861, f=i16 -3 ("t")) -> (s? t:f=w863:i16)
        n233 = Decrement(x=w854) -> (x-1=w852:i32)
        n234 = for {
          N: w852 -> [_]
          tunnel: w848 -> [w877]
          tunnel: w863 -> [w876]
          tunnel: w850 -> [w873]
          i -> [w875]
          n235 = Increment(x=w875) -> (x+1=w874:i32)
          n236 = property on="Graph" class="XYGraph (strict)"("Active Plot"=w874, "Plot.Plot Color"=w873, "Plot.Fill/Point Color"=w877, "Plot.Fill To"=w876) -> ()  [unwired: 2 in, 2 out]
        }
        n237 = property on="Graph" class="XYGraph (strict)"("Plot Area:Colors:BG Color"=w848) -> ()  [unwired: 2 in, 2 out]
        n238 = property on="Graph" class="XYGraph (strict)"("Active Plot"=u32 0, "Plot.Plot Color"=w851, "Plot.Fill To"=w855, "Active Plot"=w854, "Plot.Plot Color"=w851, "Plot.Fill To"=w855) -> ()  [unwired: 2 in, 2 out]
      }
      frame "Refresh colors" {
        n239 = Array Size(array=w884) -> (size(s)=w879:i32)
        n240 = Array Size(array=w881) -> (size(s)=w882:i32[])
        n241 = Index Array(array=w882, index=0) -> (element=w880:i32)
        n242 = Not Equal?(x=w879, y=w880) -> (x != y?=w878:bool)
        n243 = case shown="True" w878 {
          tunnel: w879 -> [_ w900]
          frame False {
          }
          frame True {
            n244 = global read "svl_Waterfall Global.vi" "colors"() -> (w897:T13)
            n245 = Decrement(x=w900) -> (x-1=w899:i32)
            n246 = Unbundle By Name(w897) -> ("frame"=w896:u32, "plot"=w895:u32)
            n247 = Decrement(x=w899) -> (x-1=w898:i32)
            n248 = for {
              N: w898 -> [_]
              tunnel: w895 -> [w901]
              i -> [w903]
              n249 = Increment(x=w903) -> (x+1=w902:i32)
              n250 = property on="Graph" class="XYGraph (strict)"("Active Plot"=w902, "Plot.Plot Color"=w901) -> ()  [unwired: 2 in, 2 out]
            }
            n251 = property on="Graph" class="XYGraph (strict)"("Active Plot"=w899, "Plot.Plot Color"=w896) -> ()  [unwired: 2 in, 2 out]
          }
        }
      }
    }
  }
